vi "Set Configuration.vi"(8 "error in (no error)":errorcluster, 10 "thread settings":T1, 11 "DSF UDP Thread Configuration in":refnum<class "UDP Thread Configuration.lvclass">=refnum) -> (0 "error out":errorcluster, 3 "DSF UDP Thread Configuration out":refnum<class "UDP Thread Configuration.lvclass">)   [LabVIEW 2020, in "UDP.lvlib" / "UDP Thread Configuration.lvclass"]
uses:
  UDP Thread Configuration.lvclass
  Thread Settings.ctl
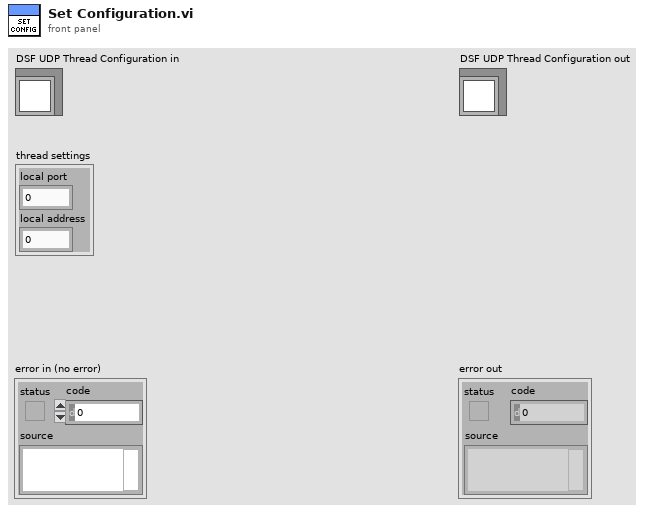
[diagram p1: front panel]
types:
  T1 = typedef "UDP.lvlib/UDP Thread Configuration.lvclass/Thread Settings.ctl" = cluster{"local port":u16, "local address":u32}
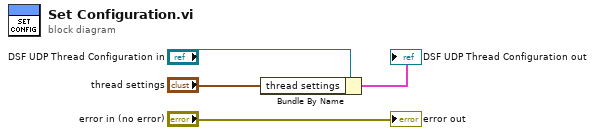
[diagram p0: block diagram]
diagram:
  n1 = Bundle By Name(cluster="DSF UDP Thread Configuration in", "thread settings"="thread settings") -> (→"DSF UDP Thread Configuration out":cluster{})
  "error out" <- "error in (no error)"
